vi "Manual Control v2.vi"() -> ()   [LabVIEW 2013]
uses:
  <vilib>/Platform/TimedLoop/XDataNode/timing_clust.ctl
  <vilib>/Platform/TimedLoop/XDataNode/nitl_modes.ctl
  <vilib>/Platform/TimedLoop/XDataNode/wakeup.ctl
  <vilib>/Instr/_visa.llb/VISA Configure Serial Port (Instr).vi
  <vilib>/Platform/TimedLoop/XDataNode/XDataNode.xnode
  <vilib>/Platform/TimedLoop/XDataNode/XDNodeRunTimeDep.lvlib
panel:
  out "Direction":string="!A"
  in  "Speed (Percent)":i32(knob) scale=0.0..100.0
  in  "Reverse":bool
  in  "Left":bool
  in  "Right":bool caption="OK Button 2"
  in  "Forward":bool
  out "write buffer":string
  in  "stop":bool
  out "error out":errorcluster
  in  "VISA resource name":refnum<visa-resource-name>
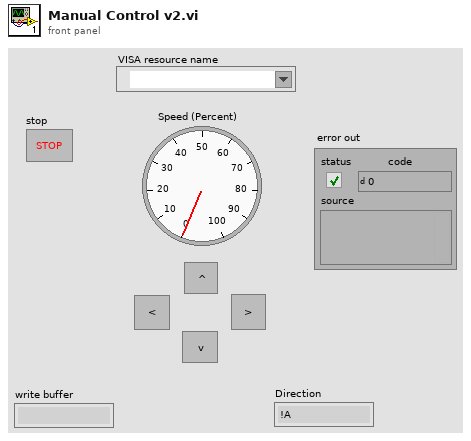
[diagram p1: front panel]
types:
  T1 = typedef "XDNodeRunTimeDep.lvlib/timing_clust.ctl" = cluster{"Expected End [f-1]":u64, "Actual End [f-1]":u64, "Finished Late? [f-1]":bool, "Expected End [i-1]":u64, "Actual End [i-1]":u64, "Finished Late? [i-1]":bool, "Expected Start [i]":u64, "Actual Start [i]":u64, "Expected Start [f]":u64, "Actual Start [f]":u64, "Source Name":string, "Structure Name":string, "Period":i64, "Deadline":i64, "Offset":i64, "Start":i64, "Priority":i32, "Timeout":i32, "Mode":T2, "Wakeup Reason":T3, "Error":errorcluster, "Source Type":string, "Secondary Source Type":string, "Global End Time":u64, "Global Start Time":u64, "Frame Duration":u64, "Iteration Duration":u64, "Assigned CPU":i32, "I/O Scan Engine Mode":u32}
  T2 = typedef "XDNodeRunTimeDep.lvlib/nitl_modes.ctl" = enum32{"No Change", "Process missed periods, maintain original phase", "Discard missed periods, maintain original phase", "Process missed periods, ignore original phase", "Discard missed periods, ignore original phase"}
  T3 = typedef "XDNodeRunTimeDep.lvlib/wakeup.ctl" = enum32{"Normal", "Aborted", "Asynchronous wakeup", "Timing source error", "Timed loop error", "Timeout"}
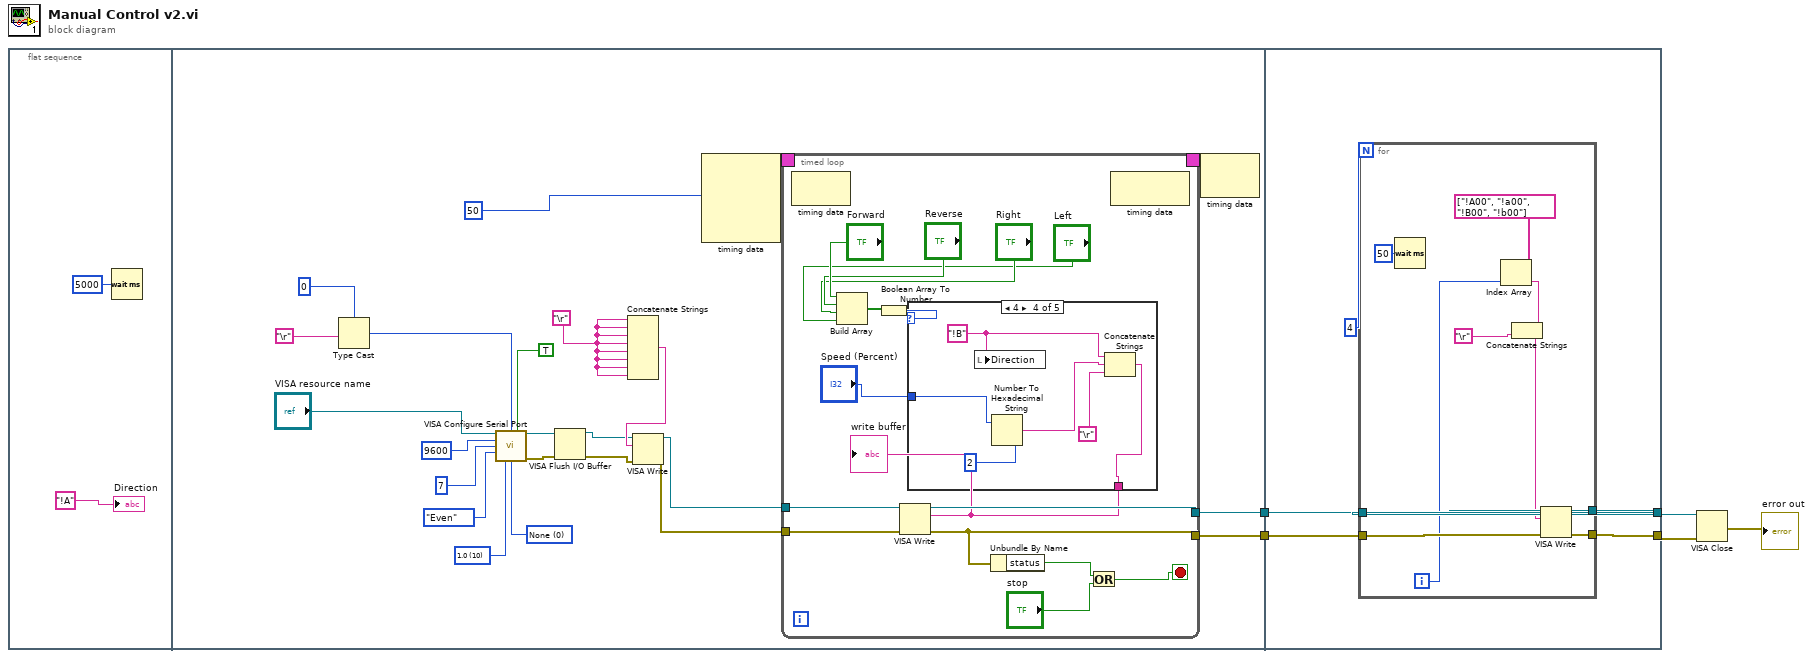
[diagram p0: block diagram]
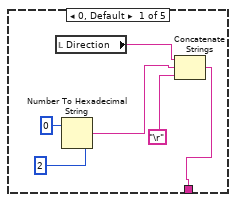
[diagram p2: hidden frame]
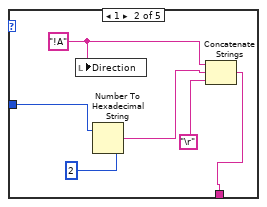
[diagram p3: hidden frame]
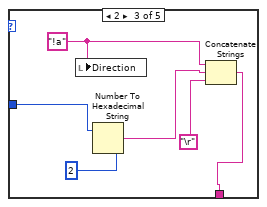
[diagram p4: hidden frame]
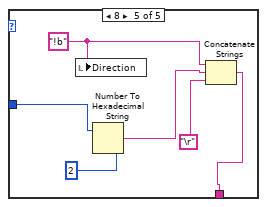
[diagram p5: hidden frame]
diagram:
  n1 = flat-sequence {
    tunnel: [w9] -> w2
    tunnel: [w8] -> w1
    tunnel: [w83] -> w4
    tunnel: [w84] -> w5
    tunnel: w2 -> [w86]
    tunnel: w1 -> [w85]
    frame #0 {
      n2 = Wait (ms)(milliseconds to wait=u32 5000) -> ()  [unwired: 1 out]
      "Direction" <- "!A" ("Direction")
    }
    frame #1 {
      w15 = "\r"
      w22 = u16 0 items=["None", "XON/XOFF", "RTS/CTS", "XON/XOFF & RTS/CTS", "DTR/DSR", "XON/XOFF & DTR/DSR"] ("flow control (0:none)")
      w23 = u16 10 items=["1.0"=10, "1.5"=15, "2.0"=20] ("stop bits (10: 1 bit)")
      n3 = Type Cast(type=0, x="\r") -> (*(type *) &x=w18:i32)
      n4 = call-poly "VISA Configure Serial Port"("VISA resource name"="VISA resource name", "termination char\n(0xA = '\\n' = LF)"=w18, "Enable Termination\nChar (T)"=TRUE ("Enable Termination\nChar (T)"), "baud rate (9600)"=u32 9600, "data bits (8)"=u16 7, "parity (0:none)"=enum16{"None", "Odd", "Even", "Mark", "Space"}."Even", "stop bits (10: 1 bit)"=w23, "flow control (0:none)"=w22) -> ("VISA resource name out"=w16:refnum<visa-resource-name>, "error out"=w17:errorcluster)  [unwired: 6 in]
      n5 = VISA Flush I/O Buffer(VISA resource name=w16, error in (no error)=w17) -> (VISA resource name out=w13:refnum<visa-resource-name>, error out=w12:errorcluster)  [unwired: 1 in]
      n6 = Concatenate Strings(w15, w15, w15, w15, w15, w15, w15, w15) -> (w14:string)
      n7 = VISA Write(VISA resource name=w13, write buffer=w14, error in (no error)=w12) -> (VISA resource name out=w11:refnum<visa-resource-name>, error out=w10:errorcluster)  [unwired: 1 out]
      n8 = node-c288(i64 50 ("Period")) -> (w30:T1)  [unwired: 3 in]
      n9 = timed-loop {
        timing: w30 -> [_]
        timing-out: [_] -> w29
        tunnel: w11 -> [w45]
        tunnel: w10 -> [w44]
        tunnel: [w39] -> w9
        tunnel: [w40] -> w8
        stop <- w41 stop-if-true
        n10 = node-c288() -> ()  [unwired: 1 in, 1 out]
        n11 = Build Array("Forward", "Reverse", "Right", "Left") -> (w34:bool[])
        n12 = Boolean Array To Number(Boolean array=w34) -> (number=w33:u32)
        n13 = case shown="4" w33 {
          tunnel: [w47 w54 w60 w66 w72] -> w31
          tunnel: "Speed (Percent)" -> [_ w53 w59 w65 w71]
          frame 0, Default {
            n14 = local read "Direction"() -> (w46:string)
            n15 = Number To Hexadecimal String(1:i16 2 ("width (-)"), 2:0 ("number")) -> (0:w51:string)
            n16 = Concatenate Strings(w46, w51, "\r") -> (w47:string)
          }
          frame 1 {
            w52 = "!A" ("string")
            n17 = local write "Direction"(w52) -> ()
            n18 = Number To Hexadecimal String(1:i16 2 ("width (-)"), 2:w53) -> (0:w57:string)
            n19 = Concatenate Strings(w52, w57, "\r") -> (w54:string)
          }
          frame 2 {
            w58 = "!a" ("string")
            n20 = local write "Direction"(w58) -> ()
            n21 = Number To Hexadecimal String(1:i16 2 ("width (-)"), 2:w59) -> (0:w63:string)
            n22 = Concatenate Strings(w58, w63, "\r") -> (w60:string)
          }
          frame 4 {
            w64 = "!B" ("string")
            n23 = local write "Direction"(w64) -> ()
            n24 = Number To Hexadecimal String(1:i16 2 ("width (-)"), 2:w65) -> (0:w69:string)
            n25 = Concatenate Strings(w64, w69, "\r") -> (w66:string)
          }
          frame 8 {
            w70 = "!b" ("string")
            n26 = local write "Direction"(w70) -> ()
            n27 = Number To Hexadecimal String(1:i16 2 ("width (-)"), 2:w71) -> (0:w75:string)
            n28 = Concatenate Strings(w70, w75, "\r") -> (w72:string)
          }
        }
        "write buffer" <- w31
        n29 = VISA Write(VISA resource name=w45, write buffer=w31, error in (no error)=w44) -> (VISA resource name out=w39:refnum<visa-resource-name>, error out=w40:errorcluster)  [unwired: 1 out]
        n30 = Unbundle By Name(w40) -> ("status"=w43:bool)
        n31 = Or(x=w43, y="stop") -> (x .or. y?=w41:bool)
        n32 = node-c288() -> ()  [unwired: 1 in, 1 out]
      }
      n33 = node-c288(w29) -> ()  [unwired: 1 out]
    }
    frame #2 {
      n34 = for {
        N: 4 -> [_]
        tunnel: w86 -> [w96]
        tunnel: w85 -> [w95]
        tunnel: [w94] -> w84
        tunnel: [w93] -> w83
        i -> [w91]
        n35 = Wait (ms)(milliseconds to wait=u32 50) -> ()  [unwired: 1 out]
        n36 = Index Array(array=string[] ["!A00", "!a00", "!B00", "!b00"], index=w91) -> (element=w89:string)
        n37 = Concatenate Strings(w89, "\r") -> (w87:string)
        n38 = VISA Write(VISA resource name=w96, write buffer=w87, error in (no error)=w95) -> (VISA resource name out=w94:refnum<visa-resource-name>, error out=w93:errorcluster)  [unwired: 1 out]
      }
    }
  }
  n39 = VISA Close(VISA resource name=w5, error in (no error)=w4) -> (error out=→"error out":errorcluster)
